vi "Parse (Delta Values).vi"(7 "Message In":string) -> (4 "DeltaAngleVector":sgl[](array[numeric]), 8 "DeltaVelocityVector":sgl[](array[numeric]), 15 "Timer":u32)   [LabVIEW 2012, in "MicroStrain 3DM-GXx.lvlib"]
doc: "Parse the data from the 0xC3 message into the Delta Angle Vector (rad) and the Delta Velocity Vector (m/s)."
uses:
  <instrlib>/MicroStrain 3DM-GXx/MicroStrain 3DM-GXx.lvlib
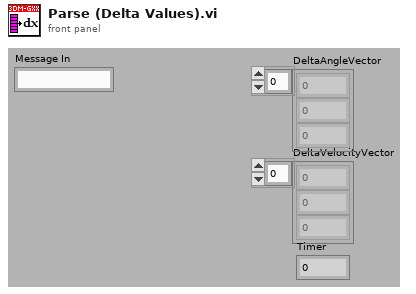
[diagram p1: front panel]
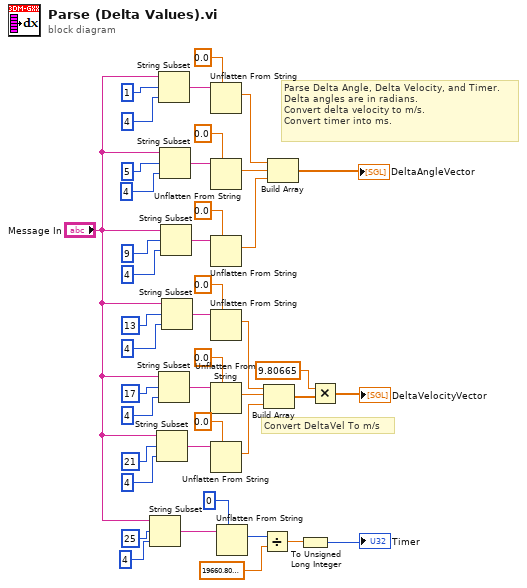
[diagram p0: block diagram]
diagram:
  # "Parse Delta Angle, Delta Velocity, and Timer.\nDelta angles are in radians.\nConvert delta velocity to m/s. \nConvert timer into ms."
  # "Convert DeltaVel To m/s"
  n1 = String Subset(string="Message In", offset (0)=25, length (rest)=4 ("length (rest)")) -> (substring=w27:string)
  n2 = String Subset(string="Message In", offset (0)=21, length (rest)=4 ("length (rest)")) -> (substring=w20:string)
  n3 = String Subset(string="Message In", offset (0)=1, length (rest)=4 ("length (rest)")) -> (substring=w40:string)
  n4 = String Subset(string="Message In", offset (0)=17, length (rest)=4 ("length (rest)")) -> (substring=w21:string)
  n5 = String Subset(string="Message In", offset (0)=5, length (rest)=4 ("length (rest)")) -> (substring=w37:string)
  n6 = String Subset(string="Message In", offset (0)=9, length (rest)=4 ("length (rest)")) -> (substring=w32:string)
  n7 = String Subset(string="Message In", offset (0)=13, length (rest)=4 ("length (rest)")) -> (substring=w26:string)
  n8 = Unflatten From String(type=sgl 0.0, binary string=w40) -> (value=w14:sgl)  [unwired: 3 in, 2 out]
  n9 = Unflatten From String(type=sgl 0.0, binary string=w37) -> (value=w13:sgl)  [unwired: 3 in, 2 out]
  n10 = Unflatten From String(type=sgl 0.0, binary string=w32) -> (value=w12:sgl)  [unwired: 3 in, 2 out]
  n11 = Unflatten From String(type=sgl 0.0, binary string=w26) -> (value=w11:sgl)  [unwired: 3 in, 2 out]
  n12 = Unflatten From String(type=sgl 0.0, binary string=w21) -> (value=w10:sgl)  [unwired: 3 in, 2 out]
  n13 = Unflatten From String(type=sgl 0.0, binary string=w20) -> (value=w9:sgl)  [unwired: 3 in, 2 out]
  n14 = Unflatten From String(type=u32 0, binary string=w27) -> (value=w6:u32)  [unwired: 3 in, 2 out]
  n15 = Divide(x=w6, y=sgl 19660.8) -> (x/y=w5:sgl)
  n16 = Build Array(w11, w10, w9) -> (w2:sgl[])
  n17 = Build Array(w14, w13, w12) -> (→"DeltaAngleVector":sgl[])
  n18 = To Unsigned Long Integer(number=w5) -> (unsigned 32bit integer=→"Timer":u32)
  n19 = Multiply(x=9.80665, y=w2) -> (x*y=→"DeltaVelocityVector":dbl[])
